vi "Swerve Wheel.vi"(7 "Wheel":T1(ring), 10 "Inputs":dbl[](array[numeric])) -> (1 "Speed":dbl, 2 "Motor Output":dbl)   [LabVIEW 2018]
uses:
  <vilib>/Rock Robotics/WPI/ThirdParty/Phoenix-LabVIEW/Motor Controller/Controls/CTRE_Phoenix_MotorControl_ControlMode.ctl
  Robot Global Data.vi
  <vilib>/addons/control/pid/pid.llb/PID (DBL).vi
  <vilib>/addons/control/pid/NI_PID_pid.lvlib
panel:
  out "PID Values":cluster{"P":dbl, "I":dbl, "D":dbl}
  # "Swerve Wheel Control\nFRC Team 34"
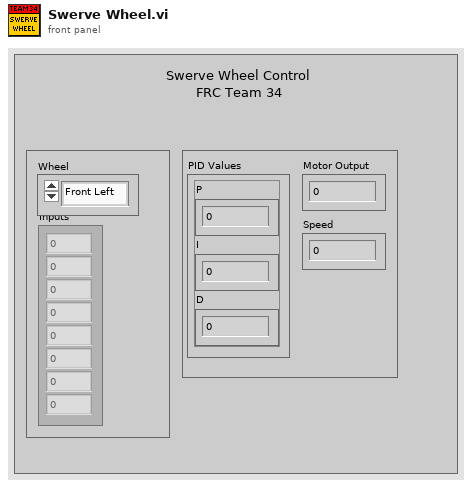
[diagram p1: front panel]
types:
  T1 = enum16{"Front Left", "Front Right", "Back Left", "Back Right"}
  T2 = cluster{"proportional gain (Kc)":dbl, "integral time (Ti, min)":dbl, "derivative time (Td, min)":dbl}
  T3 = typedef "CTRE_Phoenix_MotorControl_ControlMode.ctl" = u16
  T4 = enum16{"Z", "Y", "X", "Rot. Point X", "Rot. Point Y", "Width/2", "Max", "Length/2"}
  T5 = typedef "Offsets.ctl" = dbl[]
  T6 = typedef "WPI_MotorControlDeviceRef.ctl" = cluster{"DeviceStatus":errorcluster, "Type":T7, "PWM":cluster{"PWM Channel":T8, "DeadBand":T9}, "CAN":cluster{"Device Number":u8, "SetOutput VI Ref":variant, "GetOutput VI Ref":variant, "Enable VI Ref":variant, "Disable VI Ref":variant, "Data":variant}, "Invert":bool, "DIO PWM":cluster{"PWM \"Enable\" Channel":T8, "DIOChannel":T10, "PWM Rate":dbl}}
  T7 = typedef "WPI_MotorControlType.ctl" = enum16{"PWM", "CAN", "DIO PWM"}
  T8 = typedef "FPGA_DIOPWMChannel.ctl" = enum8{"PWM 0", "PWM 1", "PWM 2", "PWM 3", "PWM 4", "PWM 5", "PWM 6", "PWM 7", "PWM 8", "PWM 9", "PWM MXP 0", "PWM MXP 1", "PWM MXP 2", "PWM MXP 3", "PWM MXP 4", "PWM MXP 5", "PWM MXP 6", "PWM MXP 7", "PWM MXP 8", "PWM MXP 9", "Invalid"}
  T9 = typedef "WPI_PWMDeadband.ctl" = cluster{"Name":string, "maxPositivePwm":i32, "minPositivePwm":i32, "centerPwm":i32, "maxNegativePwm":i32, "minNegativePwm":i32, "angularRange":u16}
  T10 = typedef "FPGA_DIOChannel.ctl" = enum8{"DIO 0", "DIO 1", "DIO 2", "DIO 3", "DIO 4", "DIO 5", "DIO 6", "DIO 7", "DIO 8", "DIO 9", "DIO MXP 0", "DIO MXP 1", "DIO MXP 2", "DIO MXP 3", "DIO MXP 4", "DIO MXP 5", "DIO MXP 6", "DIO MXP 7", "DIO MXP 8", "DIO MXP 9", "DIO MXP 10", "DIO MXP 11", "DIO MXP 12", "DIO MXP 13", "DIO MXP 14", "DIO MXP 15", "SPI Port CS1", "SPI Port CS2", "SPI Port CS3", "SPI Port MISO", "SPI Port MOSI", "Invalid"}
  T11 = typedef "WPI_AnalogChannelDevRef.ctl" = cluster{"DevStatus":errorcluster, "Analog Channel":T12}
  T12 = typedef "FPGA_AIChannel.ctl" = enum8{"AI 0", "AI 1", "AI 2", "AI 3", "AI MXP 0", "AI MXP 1", "AI MXP 2", "AI MXP 3", "Invalid"}
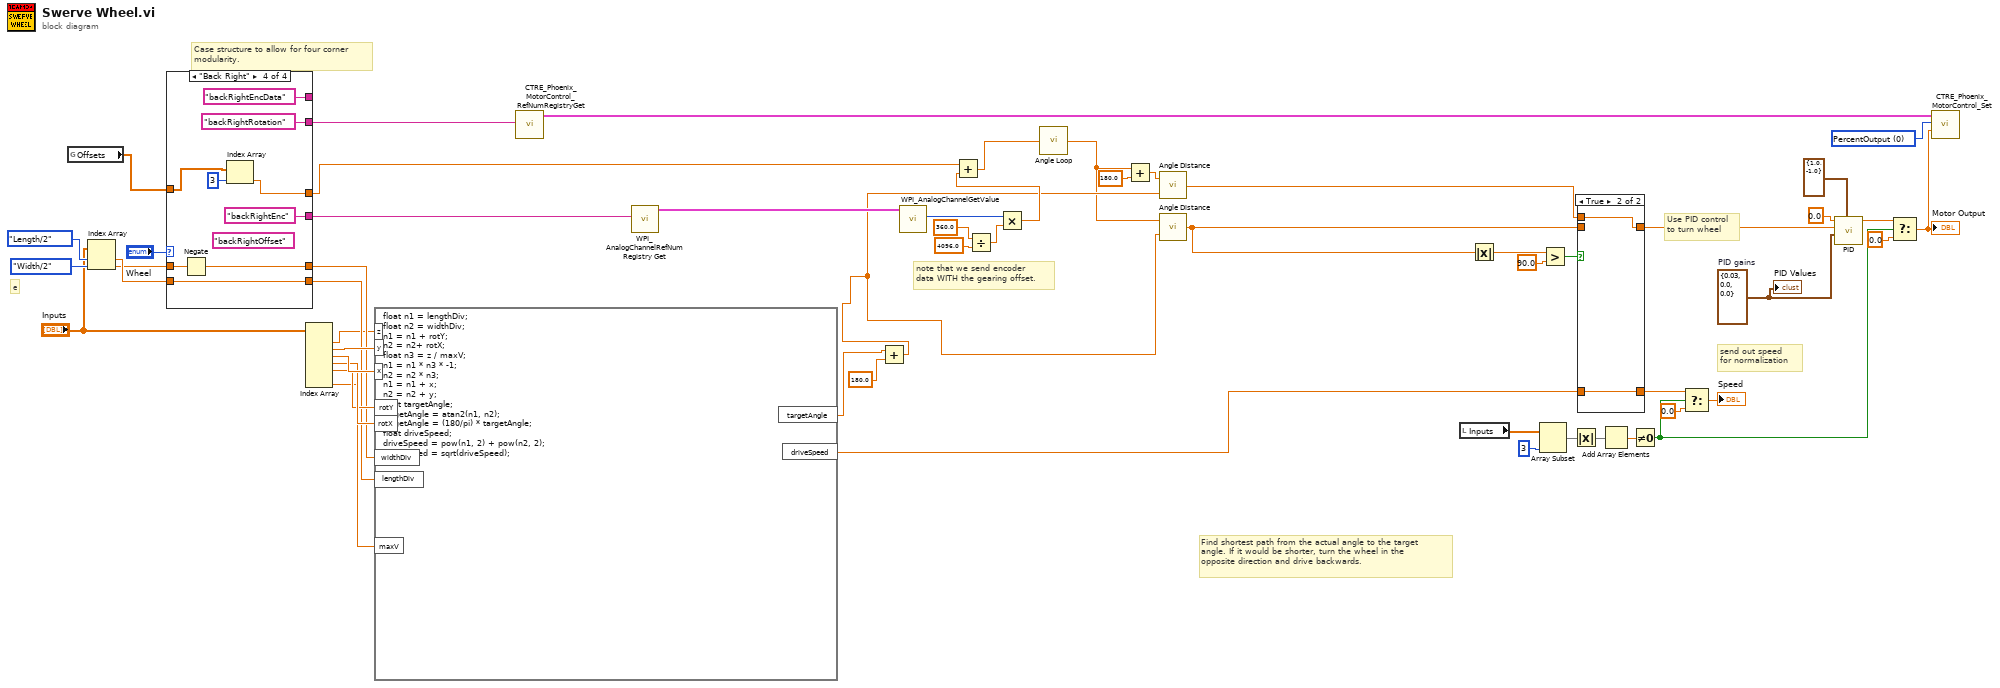
[diagram p0: block diagram]
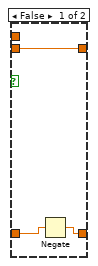
[diagram p2: hidden frame]
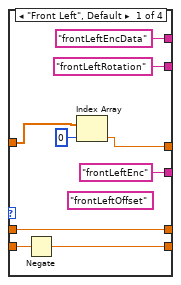
[diagram p3: hidden frame]
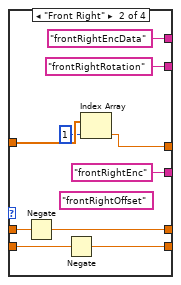
[diagram p4: hidden frame]
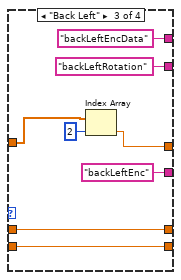
[diagram p5: hidden frame]
diagram:
  w28 = T2 {"proportional gain (Kc)"=0.03, "integral time (Ti, min)"=0.0, "derivative time (Td, min)"=0.0}  # PID gains
  w37 = T3 0 items=["PercentOutput"=0, "Position"=1, "Velocity"=2, "Current"=3, "Follower"=5, "MotionProfile"=6, "MotionMagic"=7, "MotionMagicArc"=8, "MotionProfileArc"=10, "Disabled"=15] ("Control Mode")
  # "e"
  # "note that we send encoder \ndata WITH the gearing offset."
  # "Case structure to allow for four corner\nmodularity."
  # "send out speed\nfor normalization"
  # "Use PID control\nto turn wheel"
  # "Find shortest path from the actual angle to the target angle. If it would be shorter, turn the wheel in the opposite direction and drive backwards."
  n1 = global read "Robot Global Data.vi" "Offsets"() -> (w8:T5)
  n2 = Index Array(array="Inputs", index #1=T4."Length/2", index #2=T4."Width/2") -> (element #1=w52:dbl, element #2=w51:dbl)
  n3 = case shown="\"Back Right\"" "Wheel" {
    tunnel: w52 -> [w64 w74 w82 w91]
    tunnel: w51 -> [w62 w72 w81 w90]
    tunnel: [w63 w73 w82 w91] -> w17
    tunnel: [w62 w71 w81 w89] -> w18
    tunnel: ["frontLeftRotation" "frontRightRotation" "backLeftRotation" "backRightRotation"] -> w39
    tunnel: ["frontLeftEnc" ("refnum name") "frontRightEnc" ("refnum name") "backLeftEnc" ("refnum name") "backRightEnc" ("refnum name")] -> w16
    tunnel: ["frontLeftEncData" ("Name") "frontRightEncData" ("Name") "backLeftEncData" ("Name") "backRightEncData" ("Name")] -> _
    tunnel: w8 -> [w56 w67 w75 w83]
    tunnel: [w57 w66 w76 w84] -> w6
    frame "Front Left", Default {
      (unwired) "frontLeftOffset" ("Name")
      n4 = Negate(x=w64) -> (-x=w63:dbl)
      n5 = Index Array(array=w56, index=0) -> (element=w57:dbl)
    }
    frame "Front Right" {
      (unwired) "frontRightOffset" ("Name")
      n6 = Negate(x=w72) -> (-x=w71:dbl)
      n7 = Negate(x=w74) -> (-x=w73:dbl)
      n8 = Index Array(array=w67, index=1) -> (element=w66:dbl)
    }
    frame "Back Left" {
      n9 = Index Array(array=w75, index=2) -> (element=w76:dbl)
    }
    frame "Back Right" {
      (unwired) "backRightOffset" ("Name")
      n10 = Negate(x=w90) -> (-x=w89:dbl)
      n11 = Index Array(array=w83, index=3) -> (element=w84:dbl)
    }
  }
  n12 = Index Array(array="Inputs") -> (element #1=w5:dbl, element #2=w25:dbl, element #3=w24:dbl, element #4=w23:dbl, element #5=w22:dbl, element #7=w21:dbl)  [unwired: 7 in, 1 out]
  n13 = formula code="float n1 = lengthDiv;\nfloat n2 = widthDiv;\nn1 = n1 + rotY;\nn2 = n2+ rotX;\nfloat n3 = z / maxV;\nn1 = n1 * n3 * -1;\nn2 = n2 * n3;\nn1 = n1 + x;\nn2 = n2 + y;\nfloat targetAngle;\ntargetAngle = atan2(n1, n2);\ntargetAngle = (180/pi) * targetAngle;\nfloat driveSpeed;\ndriveSpeed = pow(n1, 2) + pow(n2, 2);\ndriveSpeed = sqrt(driveSpeed);"("z"=w5, "y"=w25, "x"=w24, "rotY"=w22, "rotX"=w23, "widthDiv"=w18, "lengthDiv"=w17, "maxV"=w21) -> ("targetAngle"=w1:dbl, "driveSpeed"=w19:dbl)
  n14 = call <vilib>:"CTRE_Phoenix_MotorControl_RefNumRegistryGet.vi"("refnum name"=w39) -> ("PhoenixMotorControlDevRef"=w38:T6)  [unwired: 9 in, 1 out]
  n15 = call <vilib>:"WPI_AnalogChannelRefNum Registry Get.vi"("refnum name"=w16) -> ("AIDeviceRef"=w12:T11)  [unwired: 9 in, 1 out]
  n16 = Add(x=w1, y=180.0) -> (x+y=w4:dbl)
  n17 = call <vilib>:"WPI_AnalogChannelGetValue.vi"("AIDeviceRef"=w12) -> ("Value"=w11:i16)  [unwired: 8 in, 2 out]
  n18 = Divide(x=360.0, y=4096.0) -> (x/y=w13:dbl)
  n19 = Multiply(x=w11, y=w13) -> (x*y=w7:dbl)
  n20 = Add(x=w6, y=w7) -> (x+y=w3:dbl)
  n21 = call "Angle Loop.vi"("Input Angle"=w3) -> ("Output Angle"=w2:dbl)
  n22 = Add(x=w2, y=180.0) -> (x+y=w35:dbl)
  n23 = call "Angle Distance.vi"("Target Angle"=w4, "Current Angle"=w35) -> ("Distance"=w34:dbl)
  n24 = call "Angle Distance.vi"("Target Angle"=w4, "Current Angle"=w2) -> ("Distance"=w31:dbl)
  n25 = local read "Inputs"() -> (w47:dbl[])
  n26 = Absolute Value(x=w31) -> (abs(x)=w30:dbl)
  n27 = Array Subset(array=w47, length=3) -> (w49:dbl[])  [unwired: 1 in]
  n28 = Greater?(x=w30, y=90.0) -> (0:w32:bool)
  n29 = Absolute Value(x=w49) -> (abs(x)=w48:dbl[])
  n30 = case shown="True" w32 {
    tunnel: w31 -> [w94 _]
    tunnel: w34 -> [_ w96]
    tunnel: [w93 w95] -> w33
    tunnel: [w94 w96] -> w26
    tunnel: w19 -> [w92 w95]
    frame False {
      n31 = Negate(x=w92) -> (-x=w93:dbl)
    }
    frame True {
    }
  }
  n32 = Add Array Elements(numeric array=w48) -> (sum=w50:dbl)
  n33 = Not Equal To 0?(x=w50) -> (x != 0?=w40:bool)
  n34 = Select(t=w33, s=w40, f=0.0) -> (s? t:f=→"Speed":dbl)
  n35 = call-poly <vilib>:"PID.vi"("output range"=cluster{"output high":dbl, "output low":dbl} {"output high"=1.0, "output low"=-1.0}, "PID gains"=w28, "process variable"=w26, "setpoint"=0.0) -> ("output"=w42:dbl)  [unwired: 6 in, 1 out]
  n36 = Select(t=w42, s=w40, f=0.0) -> (s? t:f=w10:dbl)
  "Motor Output" <- w10
  n37 = call <vilib>:"CTRE_Phoenix_MotorControl_Set.vi"("Output"=w10, "Control Mode"=w37, "PhoenixMotorControlDevRef"=w38) -> ()  [unwired: 7 in, 2 out]
  "PID Values" <- w28
